vi "RYTDecode.vi"(11 "String":string) -> (3 "YTrace":dbl[](array[numeric]))   [LabVIEW 2017, in "SARemote.lvlib"]
uses:
  SARemote.lvlib
panel:
  out "output cluster":T1
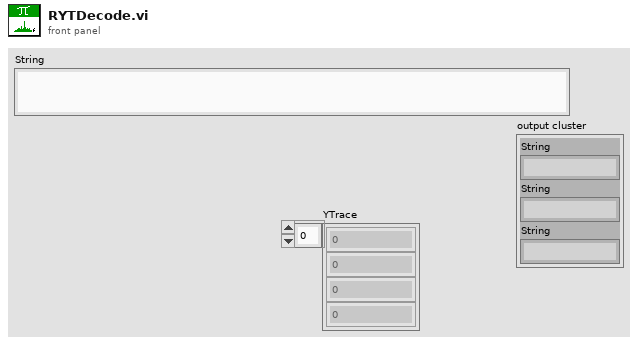
[diagram p1: front panel]
types:
  T1 = cluster{"String":string, "String":string, "String":string}
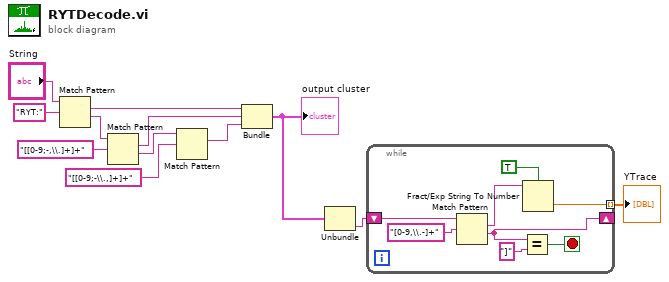
[diagram p0: block diagram]
diagram:
  n1 = Match Pattern(string="String", regular expression="RYT:") -> (match substring=w6:string, after substring=w10:string)  [unwired: 1 in, 2 out]
  n2 = Match Pattern(string=w10, regular expression="[[0-9;-,\\.]+]+") -> (match substring=w5:string, after substring=w7:string)  [unwired: 1 in, 2 out]
  n3 = Match Pattern(string=w7, regular expression="[[0-9;-\\.,]+]+") -> (match substring=w4:string)  [unwired: 1 in, 3 out]
  n4 = Bundle("String"=w6, "String"=w5, "String"=w4) -> (w1:T1)  [unwired: 1 in]
  "output cluster" <- w1
  n5 = Unbundle(w1) -> ("String"=w2:string)  [unwired: 2 out]
  n6 = while {
    shift-right: [w17] -> _
    shift-left: w2 -> [w20]
    tunnel: [w14] -> w3 mode=indexing
    stop <- w16 stop-if-true
    n7 = Match Pattern(string=w20, regular expression="[0-9,\\.-]+") -> (match substring=w15:string, after substring=w17:string)  [unwired: 1 in, 2 out]
    n8 = Equal?(x=w17, y="]") -> (x = y?=w16:bool)
    n9 = Fract/Exp String To Number(use system decimal point (T)=TRUE, string=w15) -> (number=w14:dbl)  [unwired: 2 in, 1 out]
  }
  "YTrace" <- w3
